vi "Query Option Information.vi"(0 "VISA resource name":refnum<visa-resource-name>, 11 "error in (no error)":errorcluster) -> (4 "VISA resource name out":refnum<visa-resource-name>, 6 "Total":i32, 8 "Option Information":T1(array[cluster]) {"Status" items=["On", "Off"]}, 15 "error out":errorcluster)   [LabVIEW 2020, in "Anritsu Signal Analyzer Series.lvlib"]
doc: "Queries option information."
uses:
  Anritsu Signal Analyzer Series.lvlib
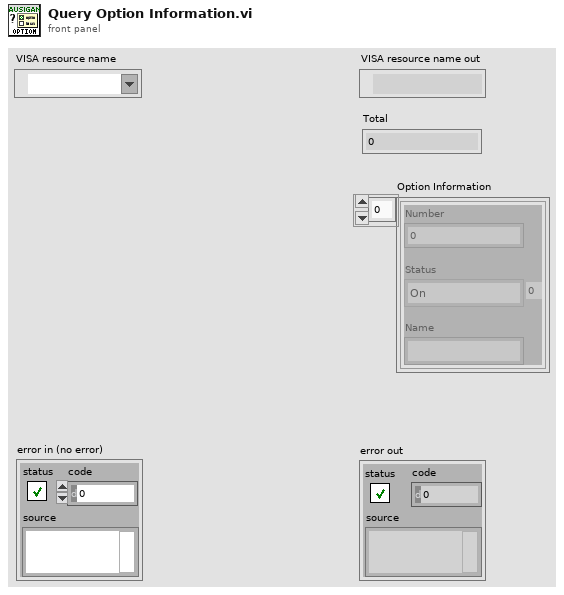
[diagram p1: front panel]
types:
  T1 = cluster{"Status":i32, "Number":i32, "Name":string}[]
  T2 = cluster{"Mode":i32, "Number":i32, "Name":string}[]
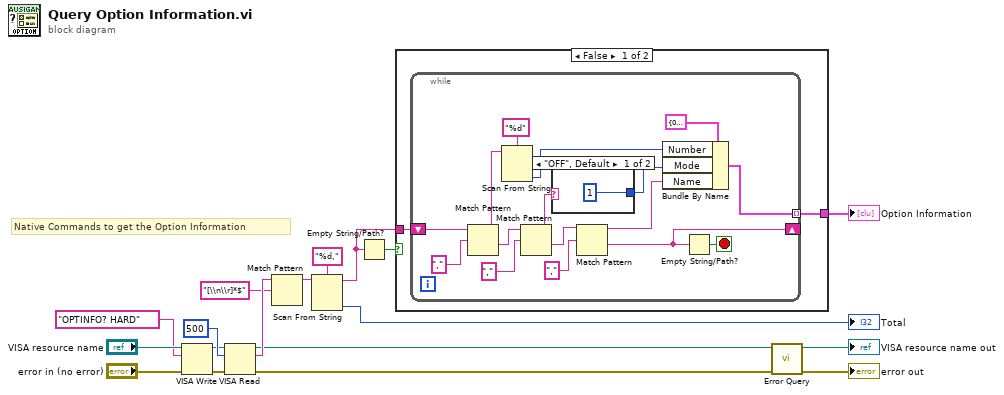
[diagram p0: block diagram]
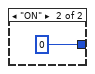
[diagram p2: hidden frame]
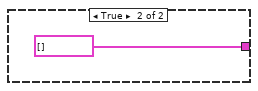
[diagram p3: hidden frame]
diagram:
  # "Native Commands to get the Option Information"
  n1 = VISA Write(VISA resource name="VISA resource name", write buffer="OPTINFO? HARD" ("_Command"), error in (no error)="error in (no error)") -> (VISA resource name out=w4:refnum<visa-resource-name>, error out=w5:errorcluster)  [unwired: 1 out]
  n2 = VISA Read(VISA resource name=w4, byte count=u32 500 ("byte count (0)"), error in (no error)=w5) -> (VISA resource name out=w2:refnum<visa-resource-name>, read buffer=w12:string, error out=w3:errorcluster)  [unwired: 1 out]
  n3 = Match Pattern(string=w12, regular expression="[\\n\\r]*$") -> (before substring=w10:string)  [unwired: 1 in, 3 out]
  n4 = Scan From String(format string="%d,", input string=w10) -> (remaining string=w11:string, output 1=→"Total":i32)  [unwired: 3 in, 2 out]
  n5 = Empty String/Path?(string/path=w11) -> (empty?=w9:bool)
  n6 = case shown="False" w9 {
    tunnel: [w20 T2 []] -> w14
    tunnel: w11 -> [w19 _]
    frame False {
      n7 = while {
        shift-right: [w30] -> _
        shift-left: w19 -> [w36]
        tunnel: [w29] -> w20 mode=indexing
        stop <- w35 stop-if-true
        n8 = Match Pattern(string=w36, regular expression=",") -> (before substring=w28:string, after substring=w34:string)  [unwired: 1 in, 2 out]
        n9 = Scan From String(format string="%d", input string=w28) -> (output 1=w27:i32)  [unwired: 3 in, 3 out]
        n10 = Match Pattern(string=w34, regular expression=",") -> (before substring=w24:string, after substring=w33:string)  [unwired: 1 in, 2 out]
        n11 = case shown="\"OFF\", Default" w24 {
          tunnel: [1 ("Return Value") 0 ("Return Value")] -> w25
          frame "OFF", Default {
          }
          frame "ON" {
          }
        }
        n12 = Match Pattern(string=w33, regular expression=",") -> (before substring=w31:string, after substring=w30:string)  [unwired: 1 in, 2 out]
        n13 = Bundle By Name(cluster=cluster{"Mode":i32, "Number":i32, "Name":string} {"Mode"=0, "Number"=0, "Name"=""} ("Option Infomation"), "Number"=w27, "Mode"=w25, "Name"=w31) -> (w29:cluster{"Mode":i32, "Number":i32, "Name":string})
        n14 = Empty String/Path?(string/path=w30) -> (empty?=w35:bool)
      }
    }
    frame True {
    }
  }
  "Option Information" <- w14
  n15 = call "Error Query.vi"("error in (no error)"=w3, "VISA resource name"=w2) -> ("error out"=→"error out":errorcluster, "VISA resource name out"=→"VISA resource name out":refnum<visa-resource-name>)  [unwired: 6 in, 2 out]
